vi "RestartProbeCycle.vi"(9 "WaferAlignment":T1, 10 "Position":i32[](array[numeric]), 11 "Array":T2(array[cluster])) -> (1 "In Starting Position":bool, 3 "Numeric":i32)   [LabVIEW 2020]
uses:
  WaferAlignmentType.ctl
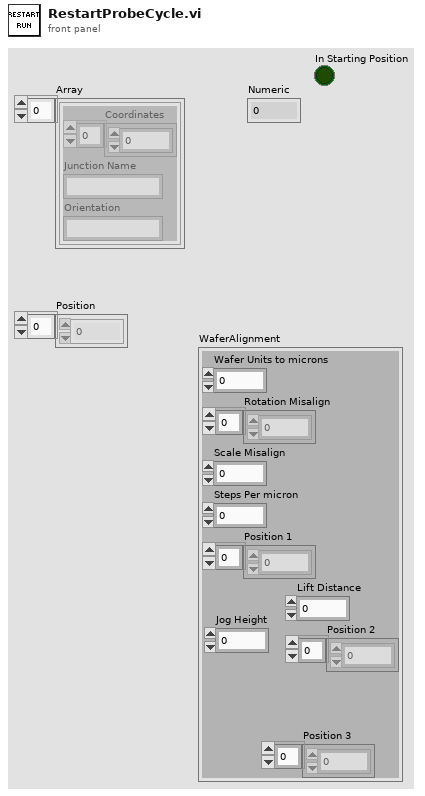
[diagram p1: front panel]
types:
  T1 = typedef "WaferAlignmentType.ctl" = cluster{"Wafer Units to microns":dbl, "Rotation Misalign":dbl[], "Scale Misalign":dbl, "Steps Per micron":dbl, "Position 1":i32[], "Position 2":i32[], "Lift Distance":i32, "Position 3":i32[], "Jog Height":i32}
  T2 = cluster{"Coordinates":dbl[], "Junction Name":string, "Orientation":string}[]
  T3 = cluster{"Coordinates":dbl[], "Junction Name":string, "Orientation":string}
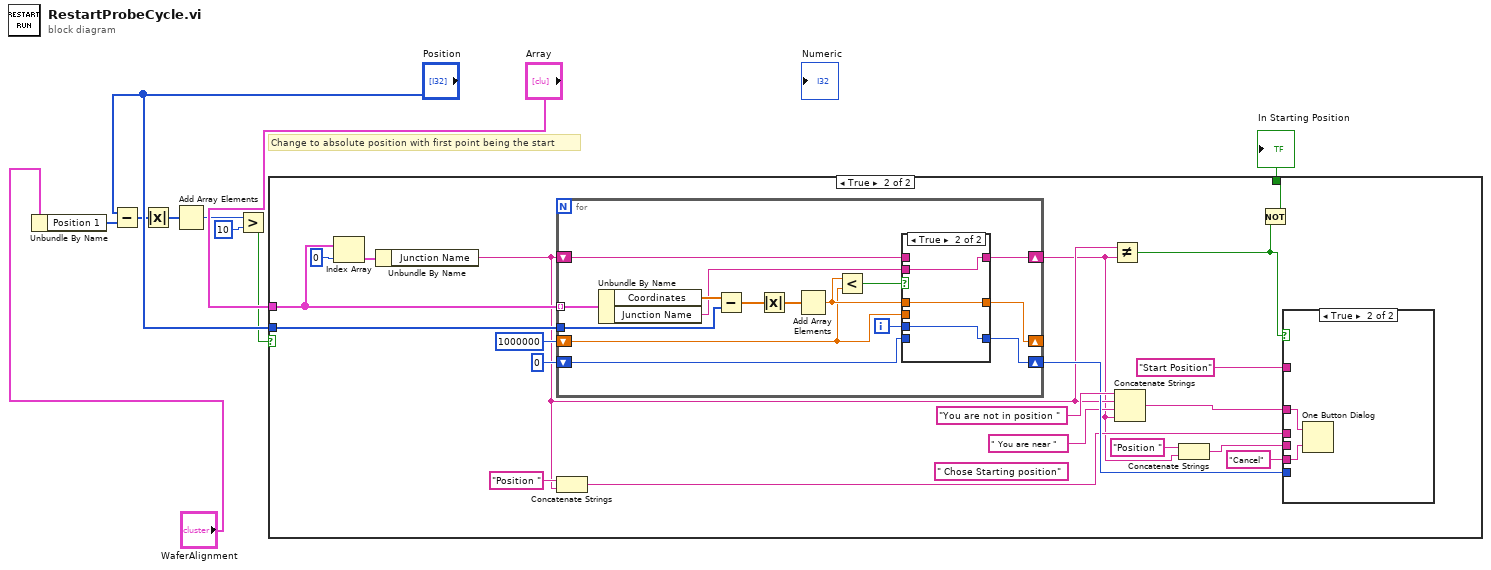
[diagram p0: block diagram]
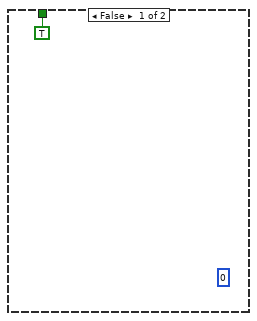
[diagram p2: hidden frame]
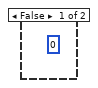
[diagram p3: hidden frame]
diagram:
  # "Change to absolute position with first point being the start"
  n1 = Unbundle By Name("WaferAlignment") -> ("Position 1"=w9:i32[])
  n2 = Subtract(x="Position", y=w9) -> (x-y=w3:i32[])
  n3 = Absolute Value(x=w3) -> (abs(x)=w4:i32[])
  n4 = Add Array Elements(numeric array=w4) -> (sum=w5:i32)
  n5 = Greater?(x=w5, y=10) -> (0:w7:bool)
  n6 = case shown="True" w7 {
    tunnel: "Array" -> [_ w23]
    tunnel: "Position" -> [_ w16]
    tunnel: [TRUE w12] -> w1
    frame False {
      (unwired) 0
    }
    frame True {
      (unwired) " Chose Starting position" ("string")
      n7 = Index Array(array=w23, index=0) -> (element=w30:T3)
      n8 = Unbundle By Name(w30) -> ("Junction Name"=w15:string)
      n9 = for {
        tunnel: w23 -> [w46] mode=indexing
        tunnel: w16 -> [w44]
        shift-right: [w38] -> w21
        shift-left: 0 -> [w37]
        shift-right: [w39] -> w14
        shift-left: w15 -> [w40]
        shift-right: [w36] -> _
        shift-left: 1000000 -> [w34]
        i -> [w41]
        n10 = Unbundle By Name(w46) -> ("Coordinates"=w45:dbl[], "Junction Name"=w43:string)
        n11 = Subtract(x=w45, y=w44) -> (x-y=w48:dbl[])
        n12 = Absolute Value(x=w48) -> (abs(x)=w47:dbl[])
        n13 = Add Array Elements(numeric array=w47) -> (sum=w35:dbl)
        n14 = Less?(x=w35, y=w34) -> (x < y?=w42:bool)
        n15 = case shown="True" w42 {
          tunnel: w43 -> [_ w54]
          tunnel: w40 -> [w51 _]
          tunnel: [w51 w54] -> w39
          tunnel: w41 -> [_ w53]
          tunnel: [w50 w53] -> w38
          tunnel: w37 -> [w50 _]
          tunnel: w34 -> [w49 _]
          tunnel: [w49 w52] -> w36
          tunnel: w35 -> [_ w52]
          frame False {
          }
          frame True {
          }
        }
      }
      n16 = Concatenate Strings("Position " ("Left Button Text (\"Yes\")"), w15) -> (w18:string)
      n17 = Not Equal?(x=w15, y=w14) -> (x != y?=w13:bool)
      n18 = Concatenate Strings("You are not in position " ("message"), w15, " You are near " ("string"), w14) -> (w27:string)
      n19 = Concatenate Strings("Position " ("string"), w14) -> (w26:string)
      n20 = Not(x=w13) -> (.not. x?=w12:bool)
      n21 = case shown="True" w13 {
        tunnel: "Cancel" ("Right Button Text (\"Cancel\")") -> [_ w33]
        tunnel: w27 -> [_ w32]
        tunnel: w26 -> [_ _]
        tunnel: "Start Position" ("Window Title (\"\")") -> [_ _]
        tunnel: w21 -> [_ _]
        tunnel: w18 -> [_ _]
        frame False {
          (unwired) 0
        }
        frame True {
          n22 = One Button Dialog(message=w32, button name ("OK")=w33) -> ()  [unwired: 1 out]
        }
      }
    }
  }
  "In Starting Position" <- w1
